vi "provide_note_book_info.vi"(8 "error in (no error)":errorcluster, 10 "notebook string in":string, 11 "GenericPlugin in":refnum<class "ScanHeadDL090202.lvclass">) -> (0 "error out":errorcluster, 2 "notebook string out":string, 3 "GenericPlugin out":refnum<class "ScanHeadDL090202.lvclass">)   [LabVIEW 2010, in "ScanHeadDL090202.lvclass"]
uses:
  ScanHeadDL090202.lvclass
  ScanHeadDL090202.lvclass/ScanHeadDL090202.ctl
  GenericScanHead/GenericScanHead/GenericScanHead.lvclass
  common/classes/ErrorController/ErrorController/class_data.vi
  common/classes/ErrorController/ErrorController/ErrorController.lvclass
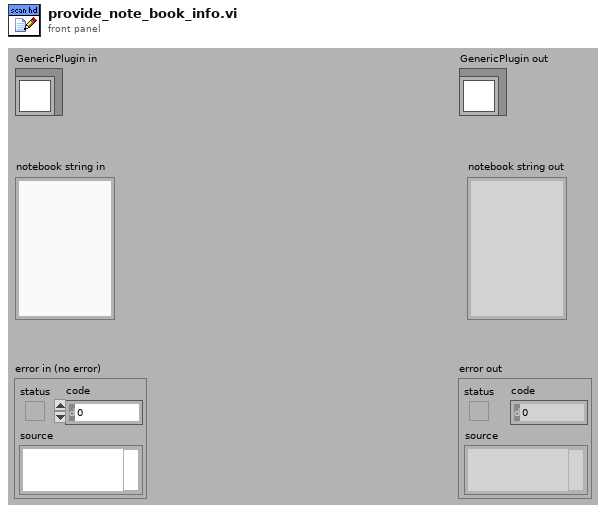
[diagram p1: front panel]
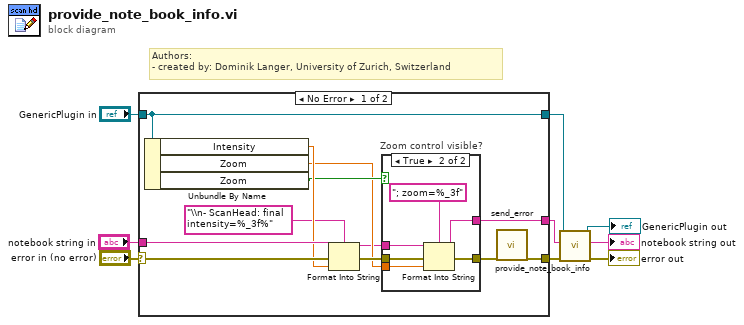
[diagram p0: block diagram]
diagram:
  # "Authors: \n- created by: Dominik Langer, University of Zurich, Switzerland"
  n1 = case shown="No Error" "error in (no error)" {
    selector: "error in (no error)" -> [w21 w32]
    tunnel: "notebook string in" -> [w20 w30]
    tunnel: "GenericPlugin in" -> [w18 w31]
    tunnel: [w19 w32] -> w3
    tunnel: [w18 w31] -> w2
    tunnel: [w11 w30] -> w1
    frame No Error {
      n2 = Unbundle By Name(w18) -> ("Intensity"=w15:dbl, "Zoom"=w13:dbl, "Zoom"=w14:bool)
      n3 = Format Into String(format string="\\n- ScanHead: final intensity=%_3f%", initial string=w20, error in=w21, w15) -> (resulting string=w12:string, error out=w17:errorcluster)
      n4 = case "Zoom control visible?" shown="True" w14 {
        tunnel: w17 -> [w23 w29]
        tunnel: [w23 w28] -> w16
        tunnel: w13 -> [_ w27]
        tunnel: w12 -> [w22 w26]
        tunnel: [w22 w25] -> w11
        frame False {
        }
        frame True {
          n5 = Format Into String(format string="; zoom=%_3f", initial string=w26, error in=w29, w27) -> (resulting string=w25:string, error out=w28:errorcluster)
        }
      }
      n6 = call "send_error.vi"("error in (no error)"=w16) -> ("error out"=w19:errorcluster)  [unwired: 10 in]
    }
    frame Error {
    }
  }
  n7 = call-parent "provide_note_book_info.vi"("error in (no error)"=w3, "notebook string in"=w1, "GenericPlugin in"=w2) -> ("error out"=→"error out":errorcluster, "notebook string out"=→"notebook string out":string, "GenericPlugin out"=→"GenericPlugin out":refnum<class "ScanHeadDL090202.lvclass">)  [unwired: 6 in]
